vi "beginACBPassPlay.vi"(8 "error in (no error)":errorcluster, 10 "Game in":refnum<class "Game.lvclass">, 11 "ACBPassPlay in":refnum<class "ACBPassPlay.lvclass">) -> (0 "error out":errorcluster, 2 "beginACBPass":bool, 3 "ACBPassPlay out":refnum<class "ACBPassPlay.lvclass">)   [LabVIEW 2020, in "ACBPassPlay.lvclass"]
uses:
  ACBPassPlay.lvclass
  Game_class/Game.lvclass
  Referee_class/command_interpreted.ctl
  Team_class/OffensivePlay.ctl
  Robot_class/roles.ctl
  Game_class/Game.lvclass/Game.ctl
  Referee_class/Referee.lvclass/Referee.ctl
  Team_class/Team.lvclass/Team.ctl
  Object_class/Object.lvclass/Object.ctl
  Object_class/Read x.vi
  Game_class/Read FieldRef.vi
  Game_class/Read OffensiveTeam.vi
  Team_class/Read RobotRef.vi
  Team_class/Read OffensivePlay.vi
  Game_class/Read Referee.vi
  Game_class/Read Utilities.lvclass.vi
  Referee_class/Read command_interpreted.vi
  Ally_class/Ally.lvclass
  C:/Users/Administrator/Desktop/SSL/SSL_AI/Team_class/Team.lvclass
  Robot_class/Robot.lvclass
  C:/Users/Administrator/Desktop/SSL/SSL_AI/Object_class/Object.lvclass
  Referee_class/Referee.lvclass
  Utilities_class/Utilities.lvclass
  Field_class/Field.lvclass
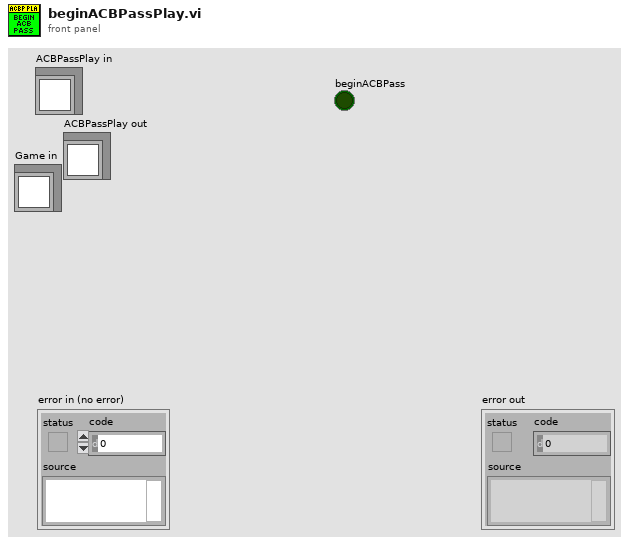
[diagram p1: front panel]
types:
  T1 = typedef "roles.ctl" = enum16{"SecondMarker", "WaitPass", "ABCThirdKicker", "ABCFirstKicker", "ABCSecondKicker", "Tabler", "TableFinalizer", "PrepareRollToPassRoller", "PrepareRollToPassReceiver", "SimplePassRoll", "SimplePassRollReceiver", "PenaltyDefense", "PreparePassReceiver 2", "PreparePassReceiver 1", "PassObserver", "Timeout", "Goto", "ZigZag", "None", "BallOutOfField", "DefenderArea", "Duelist", "AttackerStop", "FollowAttacker", "KeeperRole", "KickPenalty", "AttackerAimGoal", "AttackerBlock", "Marker", "Halt", "Shoot", "PassKicker", "PassReceiver", "TestRole", "PenaltyAttacker"}
  T2 = typedef "command_interpreted.ctl" = enum16{"Goal Ally", "Goal Enemy", "Ball Placement Enemy", "Ball Placement Ally", "Normal Half Time", "Extra Time  Break", "Extra Half Time", "None", "Post Game", "PKA Normal Start", "Prepare Kickoff Ally", "PKE Normal Start", "Prepare Kickoff Enemy", "Force Start", "Halt", "Timeout", "Prepare Penalty Ally", "Prepare Penalty Enemy", "PPA NormalStart", "PPE Normal Start", "Indirect Free Ally", "Direct Free Enemy", "Direct Free Ally", "Indirect Free Enemy", "Stop"}
  T3 = typedef "OffensivePlay.ctl" = enum16{"KeeperPassToStriker", "PrepareKeeperPass", "ACBPass", "ABCPass", "PrepareTriplePass", "TableWithStriker", "TableWith2ndStrikerPlay", "PrepareDoublePass", "PrepareRollToPass", "SimplePass", "PreparePass", "PassToStriker", "BallOutOfField", "PassTo2ndStriker", "StopOffensive", "Prepare Penalty Enemy", "EnemyPossessionAtEnemyField", "EnemyPossesionAtOurField", "TestPlay", "PreparePenaltyAlly", "KickPenaltyAlly", "PrepareKickoffAlly", "PrepareKickoffEnemy", "IndirectEnemy", "DirectEnemy", "PreparePassInGame1", "NormalGame", "DirectKick", "Pass", "Halt", "Timeout", "PassPlay", "PenaltyEnemy"}
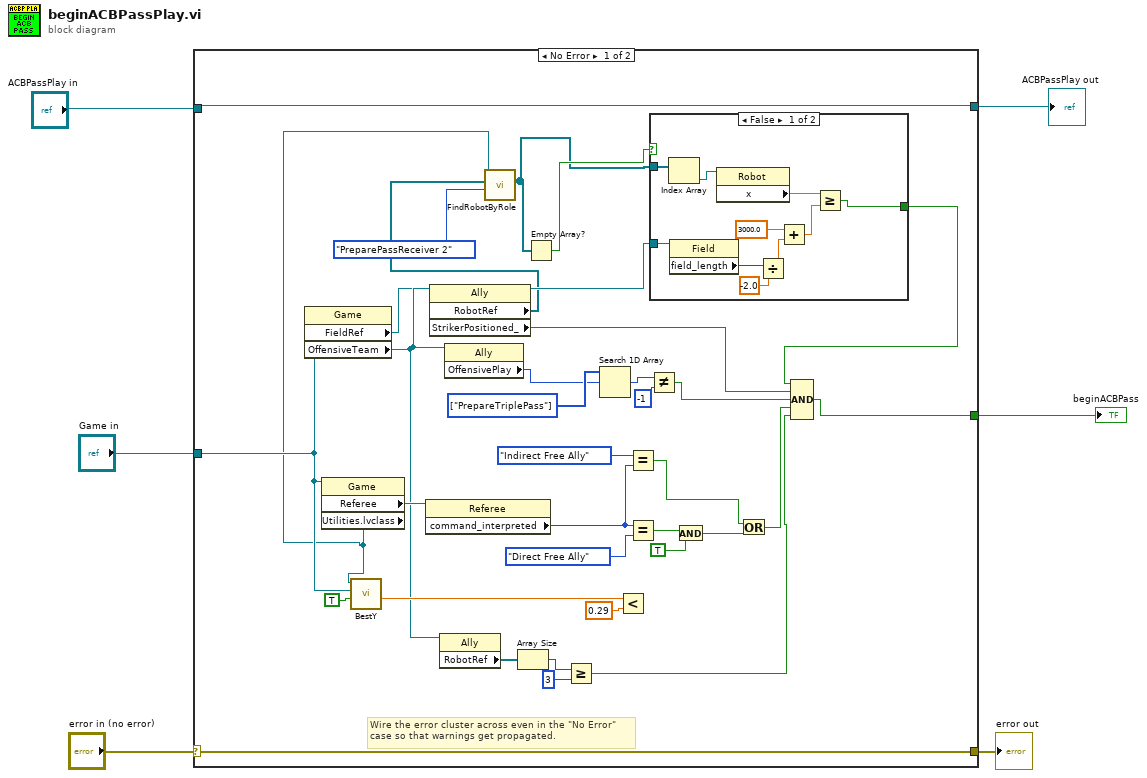
[diagram p0: block diagram]
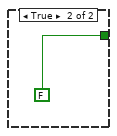
[diagram p2: hidden frame]
diagram:
  n1 = case shown="No Error" "error in (no error)" {
    selector: "error in (no error)" -> [w39 w53]
    tunnel: [w39 w53] -> w5
    tunnel: [w40 w52] -> w1
    tunnel: "ACBPassPlay in" -> [w40 w52]
    tunnel: "Game in" -> [w21 _]
    tunnel: [w20 _] -> w3
    frame No Error {
      w17 = T3[] [enum."PrepareTriplePass"] items=["KeeperPassToStriker", "PrepareKeeperPass", "ACBPass", "ABCPass", "PrepareTriplePass", "TableWithStriker", "TableWith2ndStrikerPlay", "PrepareDoublePass", "PrepareRollToPass", "SimplePass", "PreparePass", "PassToStriker", "BallOutOfField", "PassTo2ndStriker", "StopOffensive", "Prepare Penalty Enemy", "EnemyPossessionAtEnemyField", "EnemyPossesionAtOurField", "TestPlay", "PreparePenaltyAlly", "KickPenaltyAlly", "PrepareKickoffAlly", "PrepareKickoffEnemy", "IndirectEnemy", "DirectEnemy", "PreparePassInGame1", "NormalGame", "DirectKick", "Pass", "Halt", "Timeout", "PassPlay", "PenaltyEnemy"] ("Array")
      # "Wire the error cluster across even in the \"No Error\"\ncase so that warnings get propagated."
      n2 = property class="Game"(reference=w21) -> ("FieldRef"=w10:refnum<class "Field.lvclass">, "OffensiveTeam"=w23:refnum<class "Ally.lvclass">)  [unwired: 1 in, 2 out]
      n3 = property class="Game"(reference=w21) -> ("Referee"=w38:refnum<class "Referee.lvclass">, "Utilities.lvclass"=w12:refnum<class "Utilities.lvclass">)  [unwired: 1 in, 2 out]
      n4 = call "BestY.vi"("Utilities in"=w12, "Game"=w21, "inimigos"=TRUE) -> ("Gap kick"=w32:dbl)  [unwired: 2 in, 4 out]
      n5 = property class="Referee"(reference=w38) -> ("command_interpreted"=w36:T2)  [unwired: 1 in, 2 out]
      n6 = property class="Ally"(reference=w23) -> ("RobotRef"=w9:refnum<class "Robot.lvclass">[], "StrikerPositioned_"=w31:bool)  [unwired: 1 in, 2 out]
      n7 = property class="Ally"(reference=w23) -> ("RobotRef"=w26:refnum<class "Robot.lvclass">[])  [unwired: 1 in, 2 out]
      n8 = property class="Ally"(reference=w23) -> ("OffensivePlay"=w16:T3)  [unwired: 1 in, 2 out]
      n9 = call "FindRobotByRole.vi"("role"=roles."PreparePassReceiver 2", "RobotRef"=w9, "Utilities in"=w12) -> ("Robots"=w8:refnum<class "Robot.lvclass">[])  [unwired: 6 in, 2 out]
      n10 = Array Size(array=w26) -> (size(s)=w25:i32)
      n11 = Empty Array?(array=w8) -> (empty?=w11:bool)
      n12 = Greater Or Equal?(x=w25, y=3) -> (x >= y?=w22:bool)
      n13 = Search 1D Array(1D array=w17, element=w16) -> (index of element=w19:i32)  [unwired: 1 in]
      n14 = Less?(x=w32, y=0.29 ("Gap kick")) -> ()  [unwired: 1 out]
      n15 = Equal?(x=command_interpreted."Indirect Free Ally" ("command_interpreted"), y=w36) -> (x = y?=w28:bool)
      n16 = Equal?(x=w36, y=command_interpreted."Direct Free Ally" ("command_interpreted")) -> (x = y?=w30:bool)
      n17 = Not Equal?(x=w19, y=-1) -> (x != y?=w15:bool)
      n18 = case shown="False" w11 {
        tunnel: [w47 FALSE] -> w7
        tunnel: w8 -> [w50 _]
        tunnel: w10 -> [w46 _]
        frame False {
          n19 = Index Array(array=w50) -> (element=w49:refnum<class "Robot.lvclass">)  [unwired: 1 in]
          n20 = property class="Field"(reference=w46) -> ("field_length"=w45:i32)  [unwired: 1 in, 2 out]
          n21 = property class="Robot"(reference=w49) -> ("x"=w48:dbl)  [unwired: 1 in, 2 out]
          n22 = Divide(x=w45, y=-2.0) -> (x/y=w43:dbl)
          n23 = Add(x=3000.0, y=w43) -> (x+y=w42:dbl)
          n24 = Greater Or Equal?(x=w48, y=w42) -> (x >= y?=w47:bool)
        }
        frame True {
        }
      }
      n25 = And(x=w30, y=TRUE) -> (x .and. y?=w29:bool)
      n26 = Or(x=w28, y=w29) -> (x .or. y?=w27:bool)
      n27 = Compound Arithmetic op=AND(w7, w31, w15, w27, w22) -> (w20:bool)
    }
    frame Error {
    }
  }
  "error out" <- w5
  "beginACBPass" <- w3
  "ACBPassPlay out" <- w1
